vi "terminate.vi"(8 "error in (no error)":errorcluster, 11 "GenericPlugin in":refnum<class "StimulatorAK101022TCP.lvclass">) -> (0 "error out":errorcluster, 3 "GenericPlugin out":refnum<class "StimulatorAK101022TCP.lvclass">)   [LabVIEW 2010, in "StimulatorAK101022TCP.lvclass"]
doc: "The dynamic dispatch version of this VI terminates the plug-in object by releasing all of its resources."
uses:
  StimulatorAK101022TCP.lvclass
  StimulatorDL090503Scaffold/StimulatorDL090503Scaffold/StimulatorDL090503Scaffold.lvclass
  StimulatorAK101022TCP.lvclass/StimulatorAK101022TCP.ctl
  StringGenerator/GenericStringGenerator/GenericStringGenerator/GenericStringGenerator.lvclass
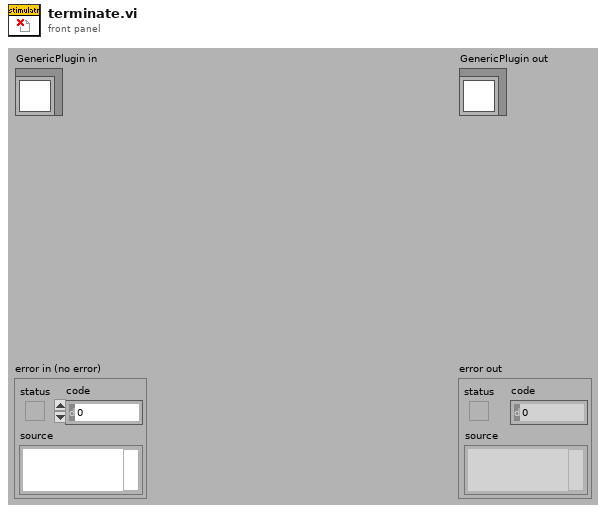
[diagram p1: front panel]
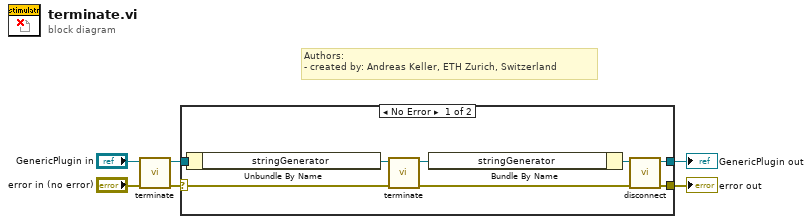
[diagram p0: block diagram]
diagram:
  # "Authors: \n- created by: Andreas Keller, ETH Zurich, Switzerland"
  n1 = call-parent "terminate.vi"("error in (no error)"="error in (no error)", "GenericPlugin in"="GenericPlugin in") -> ("error out"=w4:errorcluster, "GenericPlugin out"=w2:refnum<class "StimulatorAK101022TCP.lvclass">)  [unwired: 8 in]
  n2 = case shown="No Error" w4 {
    selector: w4 -> [w9 w16]
    tunnel: [w14 w16] -> w3
    tunnel: [w13 w15] -> w1
    tunnel: w2 -> [w7 w15]
    frame No Error {
      n3 = Unbundle By Name(w7) -> ("stringGenerator"=w11:refnum<class "GenericStringGenerator.lvclass">)
      n4 = call-dynamic "terminate.vi"("error in (no error)"=w9, "GenericPlugin in"=w11) -> ("error out"=w8:errorcluster, "GenericPlugin out"=w10:refnum<class "GenericStringGenerator.lvclass">)  [unwired: 8 in]
      n5 = Bundle By Name(cluster=w7, "stringGenerator"=w10) -> (w12:refnum<class "StimulatorAK101022TCP.lvclass">)
      n6 = call-dynamic "disconnect.vi"("error in (no error)"=w8, "StimulatorAK101022TCP in"=w12) -> ("error out"=w14:errorcluster, "StimulatorAK101022TCP out"=w13:refnum<class "StimulatorAK101022TCP.lvclass">)  [unwired: 8 in]
    }
    frame Error {
    }
  }
  "error out" <- w3
  "GenericPlugin out" <- w1
